vi "XML-String in Werte-Array.vi"(1 "XML-String":string) -> (0 "Werte":string[](array[string]))   [LabVIEW 2020, in "Anlagenuebersicht.lvlib" / "VisBx Anzeige.lvlib"]
doc: "Holt aus dem XML-String einer Umgebungsvariablen, der einen flachen Cluster zur Prozesskopplung enthält, die Werte aller Prozessvariablen."
uses:
  VisBx Anzeige.lvlib
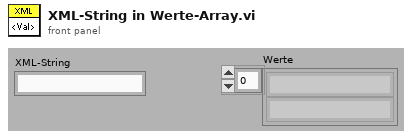
[diagram p1: front panel]
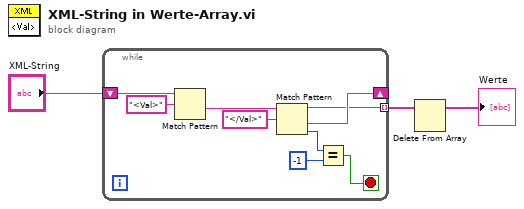
[diagram p0: block diagram]
diagram:
  n1 = while {
    shift-right: [w8] -> _
    shift-left: "XML-String" -> [w10]
    tunnel: [w7] -> w2 mode=indexing
    stop <- w4 stop-if-true
    n2 = Match Pattern(string=w10, regular expression="<Val>") -> (after substring=w9:string)  [unwired: 4 out]
    n3 = Match Pattern(string=w9, regular expression="</Val>") -> (before substring=w7:string, after substring=w8:string, offset past match=w6:i32)  [unwired: 2 out]
    n4 = Equal?(x=w6, y=-1) -> (x = y?=w4:bool)
  }
  n5 = Delete From Array(array=w2) -> (array with subset deleted=→"Werte":string[])  [unwired: 2 in, 1 out]
